vi "combineAudioAndVideo.vi"(8 "error in (no error)":errorcluster, 10 "Video path":path, 11 "Audio path":path) -> (0 "error out":errorcluster, 1 "return code":i32)   [LabVIEW 2017]
doc: "Invoke ffmpeg to combine audio and video files into a single .avi file.\n\nRequires that ffmpeg be installed on the system."
panel:
  out "resulting string":string
  out "Post system call error":errorcluster
  out "standard output":string
  out "standard error":string
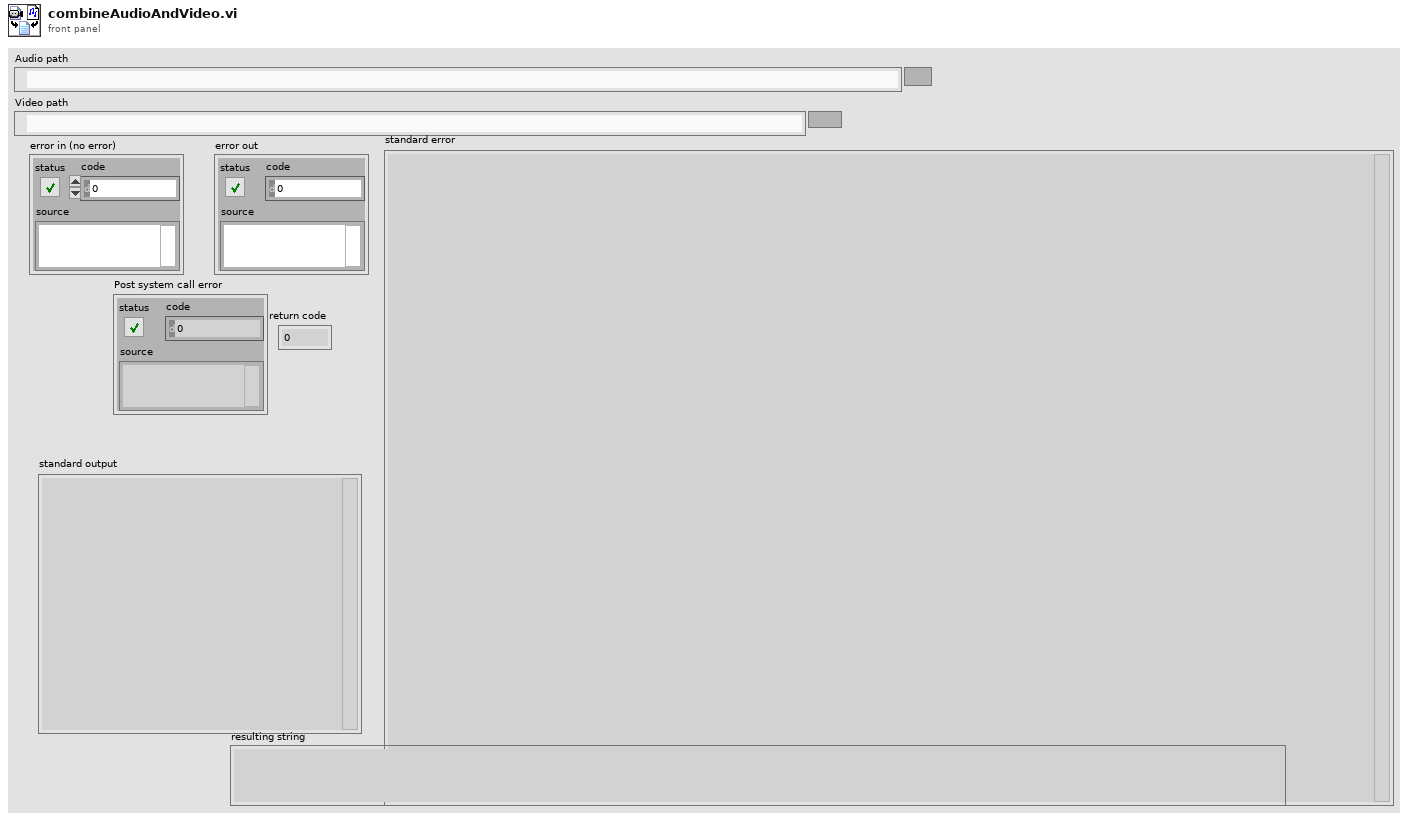
[diagram p1: front panel]
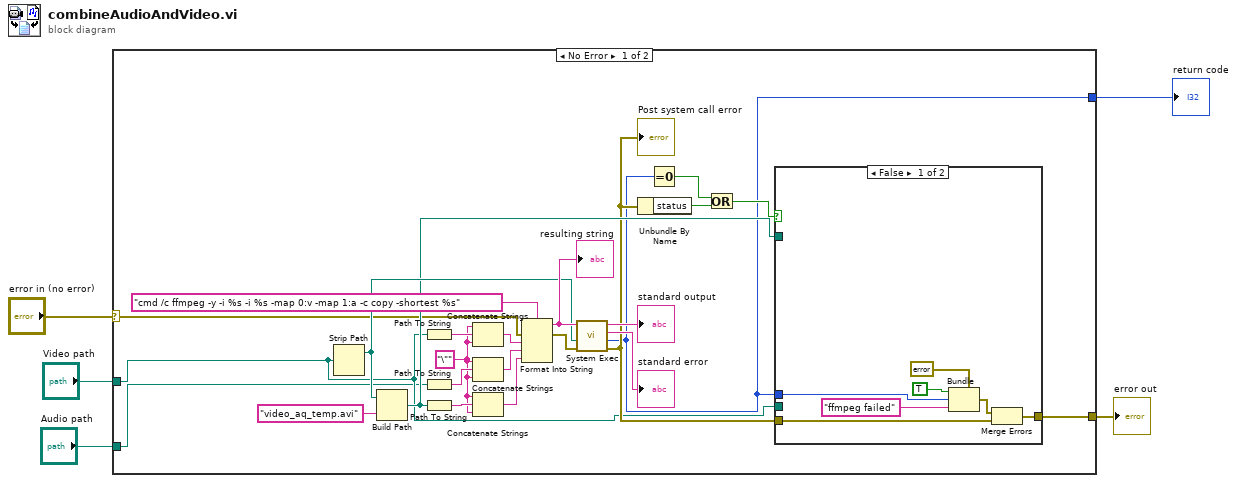
[diagram p0: block diagram]
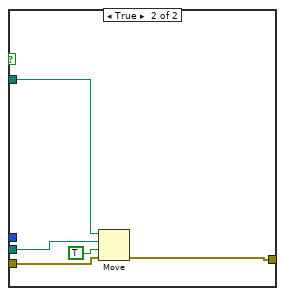
[diagram p2: hidden frame]
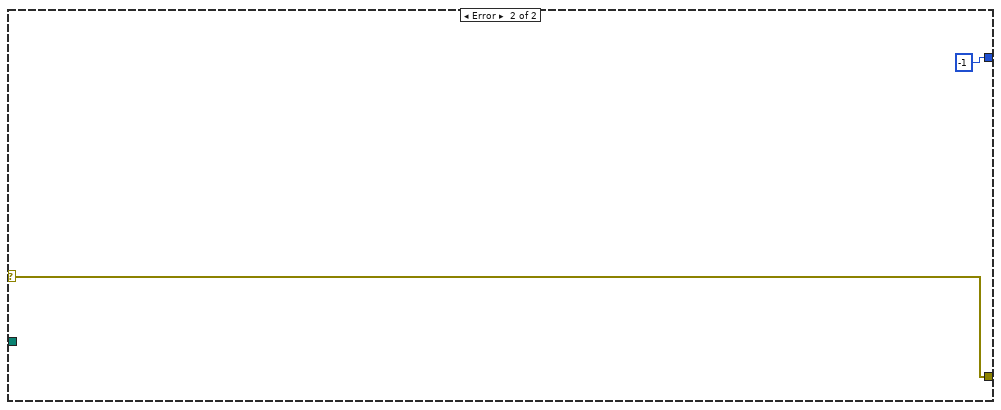
[diagram p3: hidden frame]
diagram:
  n1 = case shown="No Error" "error in (no error)" {
    selector: "error in (no error)" -> [w11 w43]
    tunnel: [w10 w43] -> w4
    tunnel: "Video path" -> [w8 _]
    tunnel: "Audio path" -> [w7 _]
    tunnel: [w6 -1 ("return code")] -> w1
    frame No Error {
      w12 = "\"" ("string")
      n2 = Strip Path(path=w8) -> (stripped path=w20:path)  [unwired: 1 out]
      n3 = Build Path(base path=w20, name or relative path="video_aq_temp.avi") -> (appended path=w18:path)
      n4 = Path To String(path=w8) -> (string=w25:string)
      n5 = Path To String(path=w7) -> (string=w26:string)
      n6 = Path To String(path=w18) -> (string=w14:string)
      n7 = Concatenate Strings(w12, w25, w12) -> (w21:string)
      n8 = Concatenate Strings(w12, w26, w12) -> (w22:string)
      n9 = Concatenate Strings(w12, w14, w12) -> (w13:string)
      n10 = Format Into String(format string="cmd /c ffmpeg -y -i %s -i %s -map 0:v -map 1:a -c copy -shortest %s" ("command line"), error in=w11, w21, w22, w13) -> (resulting string=w29:string, error out=w28:errorcluster)  [unwired: 1 in]
      "resulting string" <- w29
      n11 = call <vilib>:"System Exec.vi"("error in (no error)"=w28, "working directory"=w20, "command line"=w29) -> ("error out"=w17:errorcluster, "return code"=w6:i32, "standard error"=→"standard error":string, "standard output"=→"standard output":string)  [unwired: 5 in]
      "Post system call error" <- w17
      n12 = Unbundle By Name(w17) -> ("status"=w15:bool)
      n13 = Equal To 0?(x=w6) -> (x = 0?=w9:bool)
      n14 = Or(x=w9, y=w15) -> (x .or. y?=w16:bool)
      n15 = case shown="False" w16 {
        tunnel: w17 -> [w30 w39]
        tunnel: w18 -> [_ w41]
        tunnel: w8 -> [_ w38]
        tunnel: [w31 w37] -> w10
        tunnel: w6 -> [w34 _]
        frame False {
          n16 = Bundle(cluster=errorcluster {"status"=FALSE, "code"=0, "source"=""} ("error out"), "status"=TRUE, "code"=w34, "source"="ffmpeg failed") -> (w36:errorcluster)
          n17 = Merge Errors(w36, w30) -> (w31:errorcluster)
        }
        frame True {
          n18 = Move(source path=w41, error in=w39, 9:TRUE ("overwrite (F)"), 10:w38) -> (error out=w37:errorcluster)  [unwired: 1 in, 2 out]
        }
      }
    }
    frame Error {
    }
  }
  "error out" <- w4
  "return code" <- w1
